vi "Determine Warnings VI.vi"() -> ()   [LabVIEW 2014]
panel:
  out "Warning?":bool
  out "Warning Text":string
  in  "Min Temp":dbl
  in  "Max Temp":dbl
  in  "Current Temp":dbl
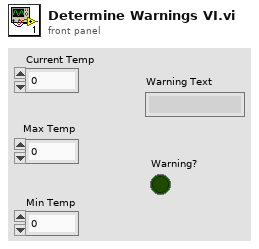
[diagram p1: front panel]
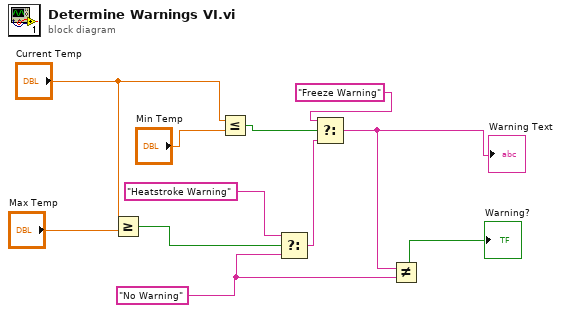
[diagram p0: block diagram]
diagram:
  w4 = "No Warning" ("String")
  n1 = Greater Or Equal?(x="Current Temp", y="Max Temp") -> (x >= y?=w11:bool)
  n2 = Less Or Equal?(x="Current Temp", y="Min Temp") -> (x <= y?=w8:bool)
  n3 = Select(t="Heatstroke Warning" ("String"), s=w11, f=w4) -> (s? t:f=w3:string)
  n4 = Select(t="Freeze Warning" ("String"), s=w8, f=w3) -> (s? t:f=w5:string)
  "Warning Text" <- w5
  n5 = Not Equal?(x=w5, y=w4) -> (x != y?=→"Warning?":bool)
